vi "Eat.vi"(8 "error in (no error)":errorcluster, 10 "String":string, 11 "Animal in":refnum<class "Animal.lvclass">) -> (0 "error out":errorcluster, 2 "String 2":string, 3 "Animal out":refnum<class "Animal.lvclass">)   [LabVIEW 2018, in "Animal.lvclass"]
uses:
  Animal.lvclass
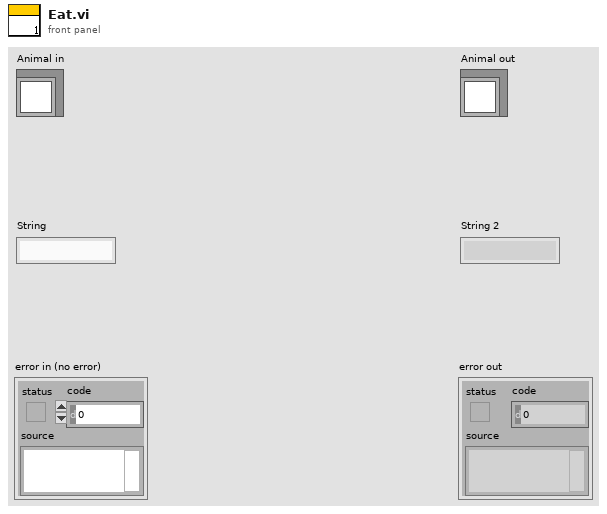
[diagram p1: front panel]
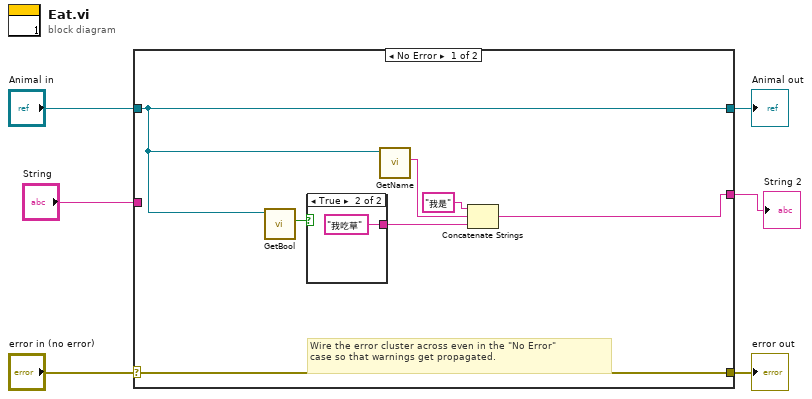
[diagram p0: block diagram]
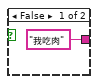
[diagram p2: hidden frame]
diagram:
  n1 = case shown="No Error" "error in (no error)" {
    selector: "error in (no error)" -> [w13 w18]
    tunnel: [w13 w18] -> w5
    tunnel: [w7 w17] -> w3
    tunnel: "Animal in" -> [w7 w17]
    tunnel: [w11 w16] -> w2
    tunnel: "String" -> [_ w16]
    frame No Error {
      # "Wire the error cluster across even in the \"No Error\"\ncase so that warnings get propagated."
      n2 = call "GetBool.vi"("Animal in"=w7) -> ("Bool"=w8:bool)  [unwired: 8 in, 2 out]
      n3 = case shown="True" w8 {
        tunnel: ["我吃肉" "我吃草"] -> w10
        frame False {
        }
        frame True {
        }
      }
      n4 = call "GetName.vi"("Animal in"=w7) -> ("Name"=w9:string)  [unwired: 8 in, 2 out]
      n5 = Concatenate Strings("我是", w9, w10) -> (w11:string)
    }
    frame Error {
    }
  }
  "error out" <- w5
  "Animal out" <- w3
  "String 2" <- w2
